vi "test Receive Signal.vi"(11 "Test Case In":refnum<class "Test PCAN.lvclass">) -> (0 "error out":errorcluster, 3 "Test Case Out":refnum<class "Test PCAN.lvclass">)   [LabVIEW 2023, in "Test PCAN.lvclass"]
uses:
  Test PCAN.lvclass
  C:/Program Files/National Instruments/LabVIEW 2023/vi.lib/Astemes/LUnit/Test Case.lvclass
  PCAN.lvclass
  D:/git/HAL/HAL GOOP4/Configuration/Configuration JSON/Configuration JSON Base/CFG JSON.lvclass
  Configuration/Configuration JSON/Configuration JSON Base/CFG JSON.lvclass
  Protocols/ICAN/ICAN.lvclass
  <vilib>/Astemes/LUnit/Test Case.lvclass/Test Case.ctl
  <vilib>/JDP Science/JSONtext/Next JSON Value.vi
  <vilib>/JDP Science/JSONtext/String Subset.vi
  <vilib>/Astemes/LUnit/Append Pass Result.vi
  <vilib>/Astemes/LUnit/Append Fail Result.vi
  <vilib>/JDP Science/JSONtext/Parsing/Advance past next JSON Value (inlined COPY).vi
  <vilib>/Astemes/LUnit/Run In UI.vi
  <vilib>/JDP Science/JSONtext/Parsing/Advance past whitespace.vi
  <vilib>/JDP Science/JSONtext/Parsing/Advance past String.vi
  <vilib>/JDP Science/JSONtext/Parsing/Advance past Number.vi
  <vilib>/Utility/error.llb/Clear Errors.vi
  <vilib>/JDP Science/JSONtext/Parsing/Advance past Line Ending.vi
  <vilib>/JDP Science/JSONtext/Parsing/Parse Full Path or Item Name.vi
  <vilib>/JDP Science/JSONtext/Parsing/Advance past Array.vi
  <vilib>/JDP Science/JSONtext/Parsing/Advance past Object.vi
  <vilib>/JDP Science/JSONtext/support/Error Cluster From Code.vi
  <vilib>/JDP Science/JSONtext/Offset/Find Item Locations by Path.vi
  <vilib>/Astemes/LUnit/Test Case.lvclass
  <vilib>/JDP Science/JSONtext/JSONtext.lvlib
panel:
  out "Output":variant
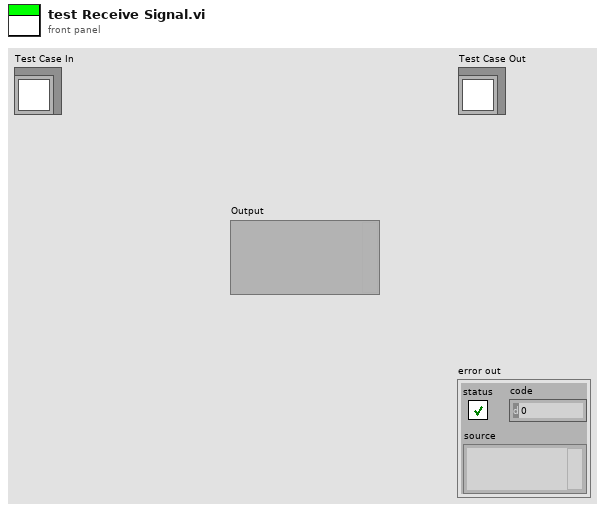
[diagram p1: front panel]
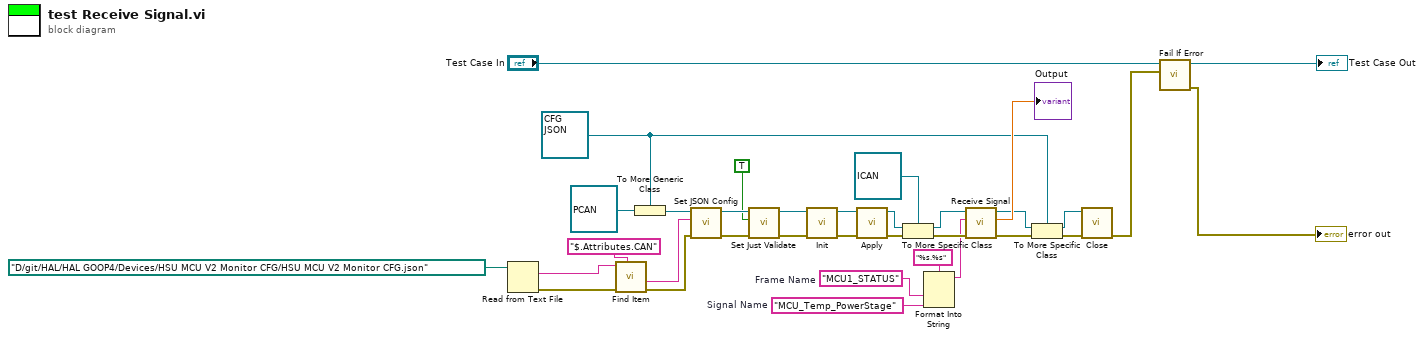
[diagram p0: block diagram]
diagram:
  w7 = "MCU1_STATUS"  # Frame Name
  w6 = "MCU_Temp_PowerStage"  # Signal Name
  w13 = refnum<class "CFG JSON.lvclass"> refnum ("HAL GOOP4.lvlib:CFG JSON.lvclass")
  n1 = Read from Text File(file (use dialog)=path "D:/git/HAL/HAL GOOP4/Devices/HSU MCU V2 Monitor CFG/HSU MCU V2 Monitor CFG.json") -> (text=w3:string, error out=w21:errorcluster)  [unwired: 3 in, 2 out]
  n2 = call <vilib>:"Find Item.vi"("$Path or Item Name"="$.Attributes.CAN", "error in (no error)"=w21, "JSON"=w3) -> ("error out"=w4:errorcluster, "<JSON>"=w2:string)  [unwired: 5 in, 2 out]
  n3 = To More Generic Class(target class=w13, reference=refnum<class "PCAN.lvclass"> refnum ("PCAN.lvclass")) -> (generic class reference=w29:refnum<class "CFG JSON.lvclass">)
  n4 = call "Set JSON Config.vi"("error in (no error)"=w4, "<JSON>Config>"=w2, "CFG Base in"=w29) -> ("error out"=w28:errorcluster, "CFG Base out"=w27:refnum<class "CFG JSON.lvclass">)  [unwired: 7 in]
  n5 = call "Set Just Validate.vi"("Just Validate"=TRUE, "CFG JSON Base in"=w27) -> ("CFG JSON Base out"=w25:refnum<class "CFG JSON.lvclass">)  [unwired: 9 in]
  n6 = call-dynamic "Init.vi"("error in"=w28, "IConfigure in"=w25) -> ("error out"=w26:errorcluster, "IConfigure out"=w23:refnum<class "CFG JSON.lvclass">)  [unwired: 8 in]
  n7 = call-dynamic "Apply.vi"("error in"=w26, "IConfigure in"=w23) -> ("error out"=w20:errorcluster, "IConfigure out"=w18:refnum<class "CFG JSON.lvclass">)  [unwired: 8 in]
  n8 = To More Specific Class(target class=refnum<class "ICAN.lvclass"> refnum ("ICAN.lvclass"), reference=w18, error in=w20) -> (specific class reference=w16:refnum<class "ICAN.lvclass">, error out=w19:errorcluster)
  n9 = Format Into String(format string="%s.%s", w7, w6) -> (resulting string=w5:string)  [unwired: 2 in, 1 out]
  n10 = call-dynamic "Receive Signal.vi"("error in"=w19, "Frame.Signal"=w5, "ICommunicate in"=w16) -> ("error out"=w12:errorcluster, "Value"=→"Output":dbl, "ICommunicate out"=w10:refnum<class "ICAN.lvclass">)  [unwired: 6 in]
  n11 = To More Specific Class(target class=w13, reference=w10, error in=w12) -> (specific class reference=w9:refnum<class "CFG JSON.lvclass">, error out=w11:errorcluster)
  n12 = call-dynamic "Close.vi"("error in"=w11, "IConfigure in"=w9) -> ("error out"=w14:errorcluster)  [unwired: 8 in, 1 out]
  n13 = call <vilib>:"Fail If Error.vi"("Assert error"=w14, "LUnit Test Case In"="Test Case In") -> ("error out"=→"error out":errorcluster, "LUnit Test Case Out"=→"Test Case Out":refnum<class "Test PCAN.lvclass">)  [unwired: 8 in]
